vi "READRX.vi"(2 "Registers to Read":u8=1, 3 "Reg. Select":u8 format="%b", 4 "SPI Config In":T1) -> (0 "Data Read":u8[](array[numeric]) format="%08b", 1 "SPI Config Out":T1)   [LabVIEW 2019]
uses:
  SPI/SPI Config.ctl
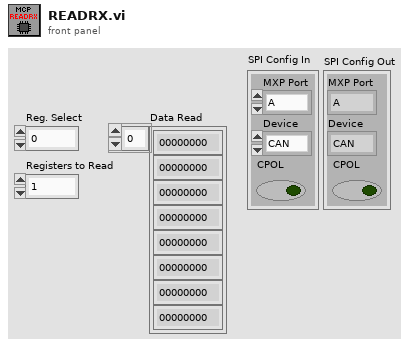
[diagram p1: front panel]
types:
  T1 = typedef "SPI Config.ctl" = cluster{"MXP Port":enum16{"A", "B"}, "Device":enum16{"CAN", "ENC", "IMU1", "IMU2"}, "CPOL":bool}
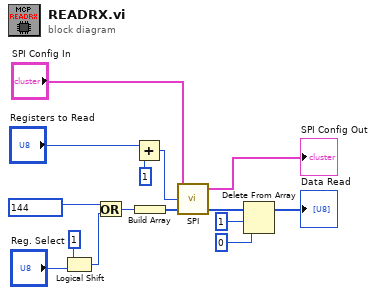
[diagram p0: block diagram]
diagram:
  n1 = Logical Shift(y=i16 1, x="Reg. Select") -> (x << y=w12:u8)
  n2 = Or(x=u8 144, y=w12) -> (x .or. y?=w11:u8)
  n3 = Add(x="Registers to Read", y=u8 1) -> (x+y=w8:u8)
  n4 = Build Array(w11) -> (w10:u8[])
  n5 = call "SPI.vi"("Data to Write"=w10, "Frames to Write"=w8, "SPI Config In"="SPI Config In") -> ("Data Read"=w4:u8[], "SPI Config Out"=→"SPI Config Out":T1)  [unwired: 1 out]
  n6 = Delete From Array(array=w4, length=1 ("index"), index=0) -> (array with subset deleted=→"Data Read":u8[])  [unwired: 1 out]
